vi "Power_Test_App.vi"(0 "millisecond multiple":u32) -> (1 "VRMS master":dbl[][](array[numeric]), 2 "Avg VRMS":dbl, 3 "IRMS Master":dbl[][](array[numeric]), 4 "Avg IRMS":dbl, 6 "Freq Master":dbl[][](array[numeric]), 8 "Avg Frequency":dbl, 10 "DCV":dbl[][](array[numeric]), 15 "Avg DCV":dbl)   [LabVIEW 2021]
uses:
  <vilib>/Waveform/WDTOps.llb/WDT Index Channel DBL.vi
  <vilib>/measure/NI_MAPro.lvlib
  <vilib>/measure/matone.llb/Extract Single Tone Information N Chan.vi
  <vilib>/measure/matone.llb/Extract Single Tone Information 1 Chan.vi
  <vilib>/measure/madcrms.llb/Basic Averaged DC-RMS for 1 Chan.vi
  <vilib>/DAQmx/read.llb/DAQmx Read (Analog 1D Wfm NChan NSamp).vi
panel:
  out "Waveform Graph":waveform(dbl)(graph)
  out "Waveform":waveform(dbl)[](graph)
  out "Elapsed Time":dbl
  out "error out":errorcluster
  out "detected frequencies":dbl[](array[numeric]) format="%.2p"
  out "DC_I":cluster{"X":dbl, "Y":dbl}[](graph)
  out "detected frequency":dbl format="%.2p"
  out "I_RMS Indicator":dbl
  out "V_RMS Indicator":dbl
  in  "stop":bool
  in  "error in":errorcluster
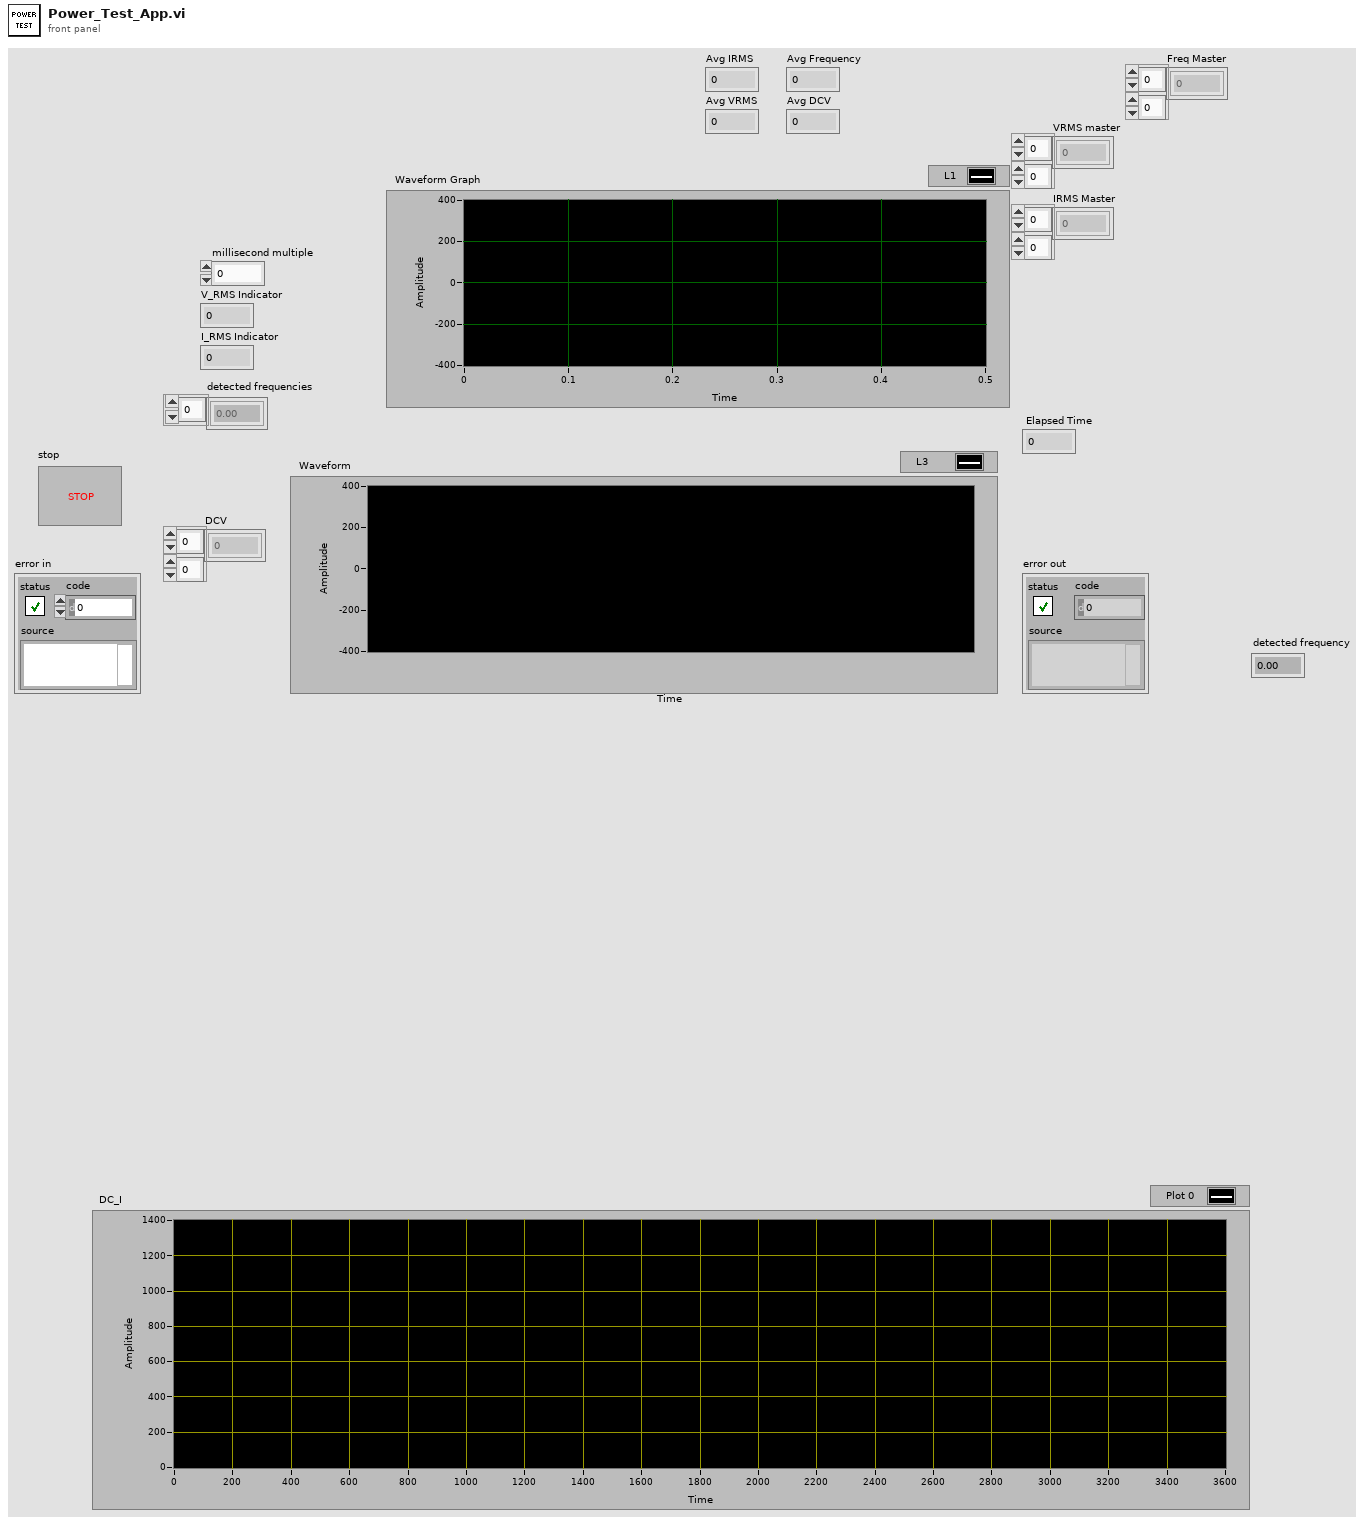
[diagram p1: front panel]
types:
  T1 = cluster{"Elapsed Time (s)":dbl, "detected frequency":dbl}
  T2 = cluster{"detected frequency":dbl, "waveform":waveform(dbl)}
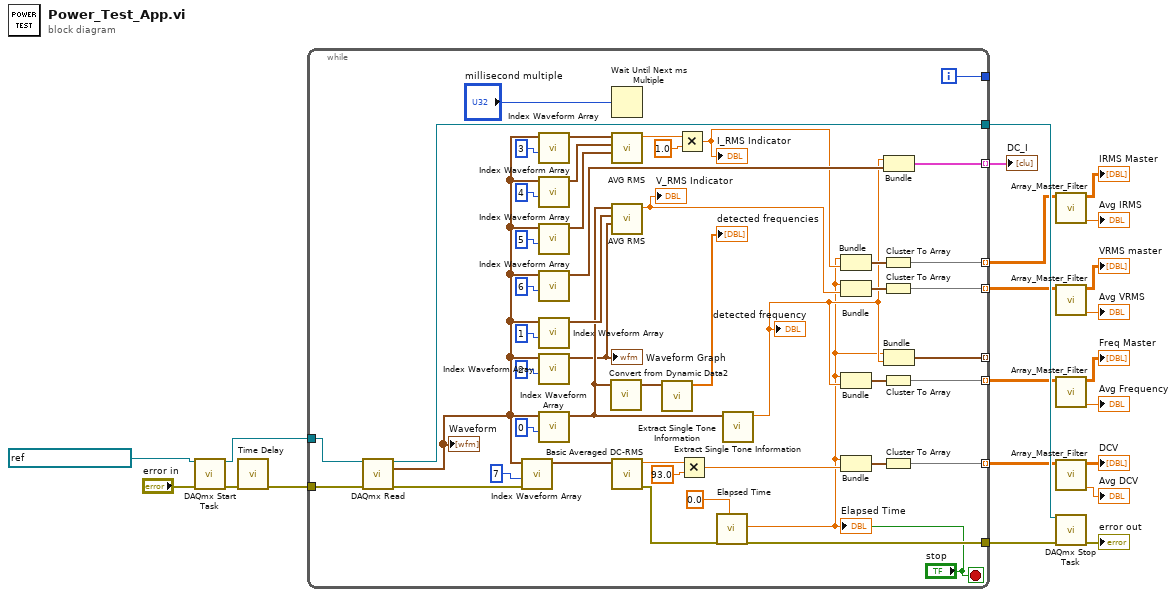
[diagram p0: block diagram]
diagram:
  n1 = call <vilib>:"DAQmx Start Task.vi"("task/channels in"=refnum<k21> "PTS_CAB1kMaster", "error in"="error in") -> ("task out"=w19:refnum<k21>, "error out"=w17:errorcluster)  [unwired: 12 in]
  n2 = call "Time Delay"("error in (no error)"=w17) -> ("error out"=w16:errorcluster)  [unwired: 10 in]
  n3 = while {
    tunnel: w19 -> [w69]
    tunnel: [w36] -> w13 mode=indexing
    tunnel: w16 -> [w49]
    tunnel: [w50] -> _ mode=indexing
    tunnel: [w47] -> w18 mode=indexing
    tunnel: [w29] -> w15
    tunnel: [w41] -> w14
    tunnel: [w40] -> w9 mode=indexing
    tunnel: [w33] -> w12 mode=indexing
    tunnel: [w32] -> _
    tunnel: [w25] -> w10 mode=indexing
    i -> [w32]
    stop <- "stop" stop-if-true
    n4 = call-poly <vilib>:"DAQmx Read.vi"("task/channels in"=w69, "error in"=w49) -> ("task out"=w41:refnum<k21>, "data"=w31:waveform(dbl)[], "error out"=w28:errorcluster)  [unwired: 11 in]
    "Waveform" <- w31
    n5 = call-poly <vilib>:"Index Waveform Array.vi"("error in (no error)"=w28, "index"=7, "waveform array"=w31) -> ("waveform"=w46:waveform(dbl))  [unwired: 7 in, 1 out]
    n6 = call-poly <vilib>:"Index Waveform Array.vi"("index"=3, "waveform array"=w31) -> ("waveform"=w57:waveform(dbl))  [unwired: 8 in, 1 out]
    n7 = call-poly <vilib>:"Index Waveform Array.vi"("index"=4, "waveform array"=w31) -> ("waveform"=w45:waveform(dbl))  [unwired: 8 in, 1 out]
    n8 = call-poly <vilib>:"Index Waveform Array.vi"("index"=5, "waveform array"=w31) -> ("waveform"=w56:waveform(dbl))  [unwired: 8 in, 1 out]
    n9 = call-poly <vilib>:"Index Waveform Array.vi"("index"=6, "waveform array"=w31) -> ("waveform"=w48:waveform(dbl))  [unwired: 8 in, 1 out]
    n10 = call-poly <vilib>:"Index Waveform Array.vi"("index"=1, "waveform array"=w31) -> ("waveform"=w59:waveform(dbl))  [unwired: 8 in, 1 out]
    n11 = call-poly <vilib>:"Index Waveform Array.vi"("index"=2, "waveform array"=w31) -> ("waveform"=w24:waveform(dbl))  [unwired: 8 in, 1 out]
    "Waveform Graph" <- w24
    n12 = call-poly <vilib>:"Index Waveform Array.vi"("index"=0, "waveform array"=w31) -> ("waveform"=w43:waveform(dbl))  [unwired: 8 in, 1 out]
    n13 = call "Convert from Dynamic Data2"("Dynamic Data Type"=w43) -> ("Array of Waveform"=w44:waveform(dbl)[])  [unwired: 3 in]
    n14 = Wait Until Next ms Multiple(millisecond multiple="millisecond multiple") -> ()  [unwired: 1 out]
    n15 = call "AVG RMS.vi"("Line 3"=w56, "Line 2"=w45, "Line 1"=w57) -> ("AVG RMS"=w55:dbl)  [unwired: 8 in]
    n16 = call "AVG RMS.vi"("Line 3"=w24, "Line 2"=w59, "Line 1"=w43) -> ("AVG RMS"=w58:dbl)  [unwired: 8 in]
    "V_RMS Indicator" <- w58
    n17 = call-poly <vilib>:"Basic Averaged DC-RMS.vi"("signal in"=w46) -> ("error out"=w30:errorcluster, "DC value"=w53:dbl)  [unwired: 7 in, 2 out]
    n18 = call-poly <vilib>:"Extract Single Tone Information.vi"("time signals in"=w44) -> ("detected frequencies"=→"detected frequencies":dbl[])  [unwired: 5 in, 5 out]
    n19 = Multiply(x=w55, y=1.0) -> (x*y=w35:dbl)
    "I_RMS Indicator" <- w35
    n20 = Multiply(x=w53, y=93.0) -> (x*y=w51:dbl)
    n21 = call "Elapsed Time"("Reset"="stop", "error in (no error)"=w30, "Set Start Time (s)"=0.0) -> ("Elapsed Time (s)"=w26:dbl, "error out"=w29:errorcluster)  [unwired: 9 in, 6 out]
    "Elapsed Time" <- w26
    n22 = call-poly <vilib>:"Extract Single Tone Information.vi"("time signal in"=w43) -> ("detected frequency"=w27:dbl)  [unwired: 5 in, 5 out]
    "detected frequency" <- w27
    n23 = Bundle("Elapsed Time (s)"=w26, w35) -> (w34:cluster{"Elapsed Time (s)":dbl, dbl})  [unwired: 1 in]
    n24 = Bundle("Elapsed Time (s)"=w26, "AVG RMS"=w58) -> (w37:cluster{"Elapsed Time (s)":dbl, "AVG RMS":dbl})  [unwired: 1 in]
    n25 = Bundle("Elapsed Time (s)"=w26, "detected frequency"=w27) -> (w38:T1)  [unwired: 1 in]
    n26 = Bundle("Elapsed Time (s)"=w26, w51) -> (w39:cluster{"Elapsed Time (s)":dbl, dbl})  [unwired: 1 in]
    n27 = Cluster To Array(cluster=w34) -> (array=w33:dbl[])
    n28 = Cluster To Array(cluster=w37) -> (array=w36:dbl[])
    n29 = Cluster To Array(cluster=w38) -> (array=w25:dbl[])
    n30 = Cluster To Array(cluster=w39) -> (array=w40:dbl[])
    n31 = Bundle("detected frequency"=w27, "waveform"=w48) -> (w47:T2)  [unwired: 1 in]
    n32 = Bundle("Elapsed Time (s)"=w26, "detected frequency"=w27) -> (w50:T1)  [unwired: 1 in]
  }
  "DC_I" <- w18
  n33 = call "Array_Master_Filter.vi"("Array in"=w12) -> ("Average"=→"Avg IRMS":dbl, "Filtered Array"=→"IRMS Master":dbl[][])  [unwired: 9 in]
  n34 = call "Array_Master_Filter.vi"("Array in"=w13) -> ("Average"=→"Avg VRMS":dbl, "Filtered Array"=→"VRMS master":dbl[][])  [unwired: 9 in]
  n35 = call "Array_Master_Filter.vi"("Array in"=w10) -> ("Average"=→"Avg Frequency":dbl, "Filtered Array"=→"Freq Master":dbl[][])  [unwired: 9 in]
  n36 = call "Array_Master_Filter.vi"("Array in"=w9) -> ("Average"=→"Avg DCV":dbl, "Filtered Array"=→"DCV":dbl[][])  [unwired: 9 in]
  n37 = call <vilib>:"DAQmx Stop Task.vi"("task/channels in"=w14, "error in"=w15) -> ("error out"=→"error out":errorcluster)  [unwired: 12 in, 1 out]
